vi "GetSetLightStatus.vi"(8 "error in":errorcluster, 9 "Light status":u8 max=1 step=1, 10 "get/set":T1=enum."set", 11 "VISA resource name":refnum<visa-resource-name>) -> (0 "error out":errorcluster, 2 "Light Status":string, 3 "VISA resource name out":refnum<visa-resource-name>)   [LabVIEW 2023, in "Thermotron 8800.lvlib"]
doc: "LGHT\nCommand name: Send or load light status\nCommand type: System status\nDescription: The query command asks the 8800 for the status of the light (on or off). The operation command allows you to remotely turn the chamber light on or off.\nSyntax: LGHT? or LGHTn\nWhere n is 0 (off) or 1 (on).\nData type: Integer\nQuery example: LGHT?\n8800 response: 1 (The chamber light is on.)\nOperation example: LGHT0\n8800 response: Turns the chamber light off."
uses:
  Thermotron 8800.lvlib
  Private/get set.ctl
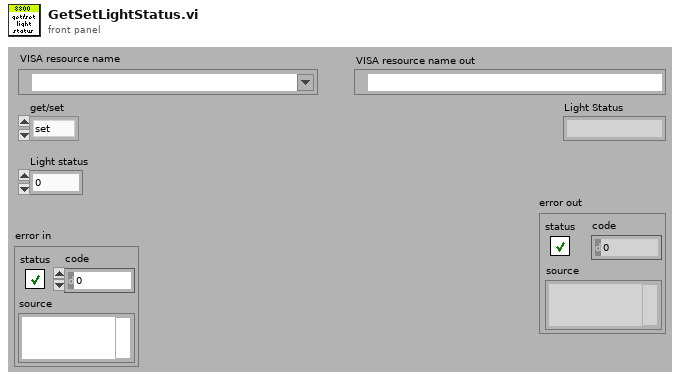
[diagram p1: front panel]
types:
  T1 = typedef "Thermotron 8800.lvlib/get set.ctl" = enum16{"get", "set"}
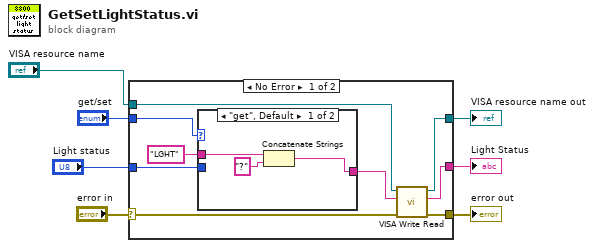
[diagram p0: block diagram]
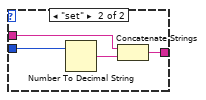
[diagram p2: hidden frame]
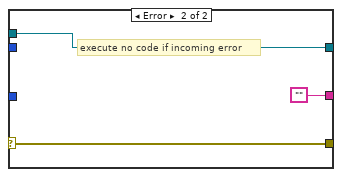
[diagram p3: hidden frame]
diagram:
  n1 = case shown="No Error" "error in" {
    selector: "error in" -> [w8 w25]
    tunnel: "get/set" -> [w16 _]
    tunnel: [w13 ""] -> w1
    tunnel: [w12 w25] -> w4
    tunnel: [w11 w26] -> w3
    tunnel: "VISA resource name" -> [w10 w26]
    tunnel: "Light status" -> [w9 _]
    frame No Error {
      n2 = case shown="\"get\", Default" w16 {
        tunnel: "LGHT" ("8800 Command") -> [w18 w23]
        tunnel: [w19 w22] -> w14
        tunnel: w9 -> [_ w20]
        frame "get", Default {
          n3 = Concatenate Strings(w18, "?" ("8800 Command")) -> (w19:string)
        }
        frame "set" {
          n4 = Number To Decimal String(number=w20) -> (decimal integer string=w21:string)  [unwired: 1 in]
          n5 = Concatenate Strings(w23, w21) -> (w22:string)
        }
      }
      n6 = call "VISA Write Read.vi"("error in (no error)"=w8, "8800 Command"=w14, "VISA Refnum in"=w10) -> ("error out"=w12:errorcluster, "read buffer"=w13:string, "VISA Refnum out"=w11:refnum<visa-resource-name>)  [unwired: 6 in]
    }
    frame Error {
      # "execute no code if incoming error"
    }
  }
  "VISA resource name out" <- w3
  "error out" <- w4
  "Light Status" <- w1
